vi "ma_Tone estimation subroutine G(f).vi"   [LabVIEW 2020, in "NI_MAPro.lvlib"]
uses:
  NI_MAPro.lvlib
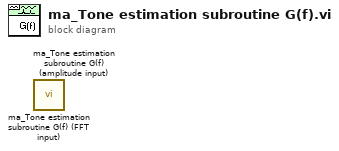
[diagram p0: block diagram]
diagram:
  n1 = call "ma_Tone estimation subroutine G(f) (FFT input).vi"() -> ()  [unwired: 5 in, 3 out]
  n2 = call "ma_Tone estimation subroutine G(f) (amplitude input).vi"() -> ()  [unwired: 6 in, 2 out]
